vi "XML-RPC Server.vi"() -> ()   [LabVIEW 2014]
doc: "This VI is an XML-RPC Server - It will accept TCP/IP client connections, interpret a properly formatted XML-RPC request, launch the LabVIEW VI mapped to that request, and return the response in XML-RPC format to the requesting connection (client). VIs called by this server must be enclosed in a VI wrapper that supports conversion of the LV arguments in to XML-RPC format and converts the LV response to XML-RPC format.\n\nThis is a single-threaded server but it will handle multiple clients with some efficiency as connection requests are queued and the requested method is launched asynchronously so pending connections do not have to wait on a previous method request to complete unless the pending connection is trying to use a method already in progress.\n\nLicense\n\nThis work is licensed under the Creative Commons Attribution 3.0 Unported License. To view a copy of this license, visit http://creativecommons.org/licenses/by/3.0/ or send a letter to Creative Commons, 171 Second Street, Suite 300, San Francisco, California, 94105, USA.\n\nMark E. Smith, Sandia National Laboratories"
uses:
  Controls/methodCall.ctl
  Controls/methodResponse.ctl
  Controls/XML-RPC Server.ctl
panel:
  out "error log file path":path
  out "method path":path
  out "Parameters":string[](array[string])
  out "error out":errorcluster
  out "methodName":string
  in  "port":u16=8080
  in  "Private Data":T3={"error"={"status"=FALSE, "code"=0, "source"=""}, "active connection ID"=refnum, "methodCall"={"methodName"="", "Parameters"=[], "connection ID"=refnum}, "methodCall queue"=refnum, "methodResponse"={"value"="", "connection ID"=refnum}, "methodResponse queue"=refnum, "Error Log File Path"=path "", "Error Log Enabled"=FALSE, "Front Panel Window:State"=enum."Hidden"}
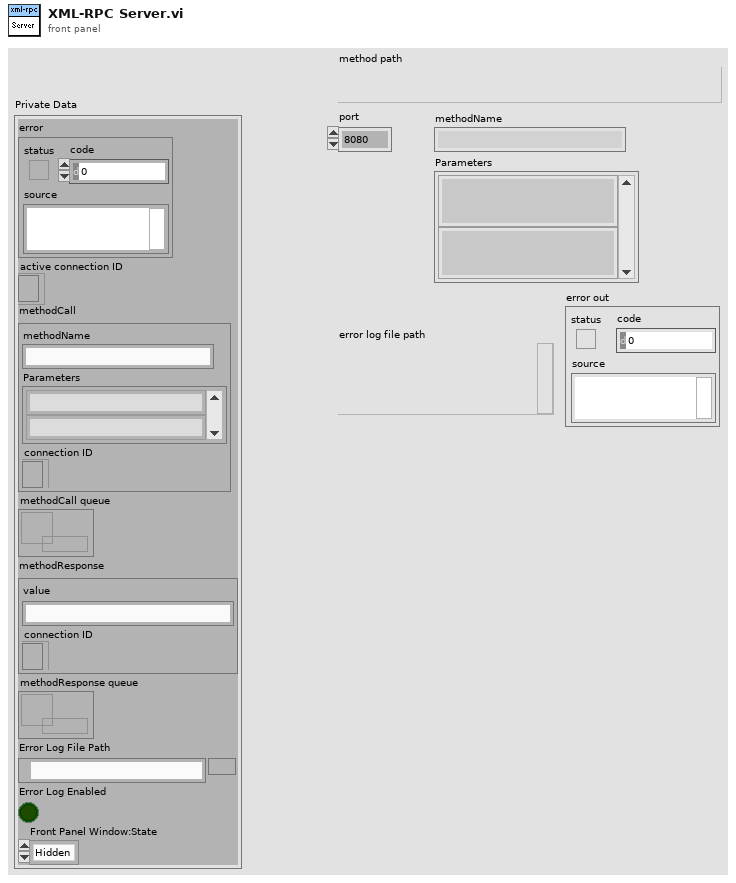
[diagram p1: front panel]
types:
  T1 = typedef "methodCall.ctl" = cluster{"methodName":string, "Parameters":string[], "connection ID":refnum<k5>}
  T2 = typedef "methodResponse.ctl" = cluster{"value":string, "connection ID":refnum<k5>}
  T3 = cluster{"error":errorcluster, "active connection ID":refnum<k5>, "methodCall":T1, "methodCall queue":refnum<queue>, "methodResponse":T2, "methodResponse queue":refnum<queue>, "Error Log File Path":path, "Error Log Enabled":bool, "Front Panel Window:State":enum32{"Invalid", "Standard", "Closed", "Hidden", "Minimized", "Maximized"}}
  T4 = typedef "XML-RPC Server.ctl" = enum16{"Initialize", "Dequeue", "Remote Procedure Call", "Server State", "Error", "Exit"}
  T5 = enum32{"Invalid", "Standard", "Closed", "Hidden", "Minimized", "Maximized"}
  T6 = enum32{"invalid app kind", "Development System", "Run Time System", "Student Edition", "Embedded LabVIEW", "Evaluation", "Custom"}
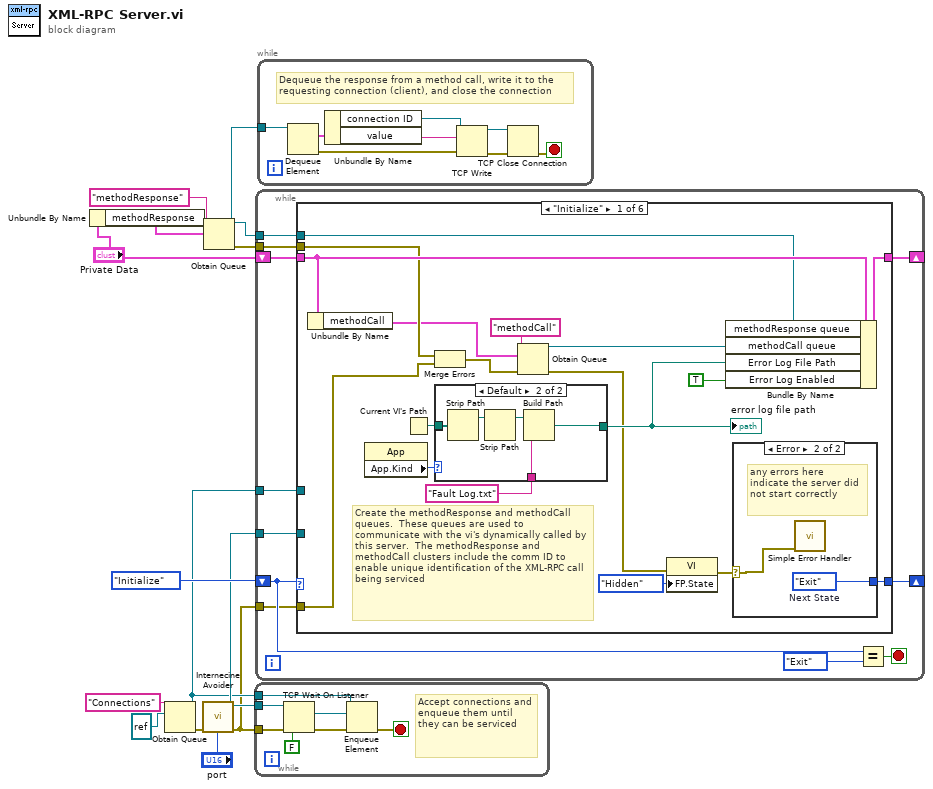
[diagram p0: block diagram]
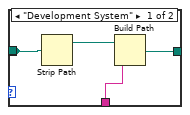
[diagram p2: hidden frame]
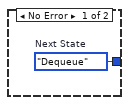
[diagram p3: hidden frame]
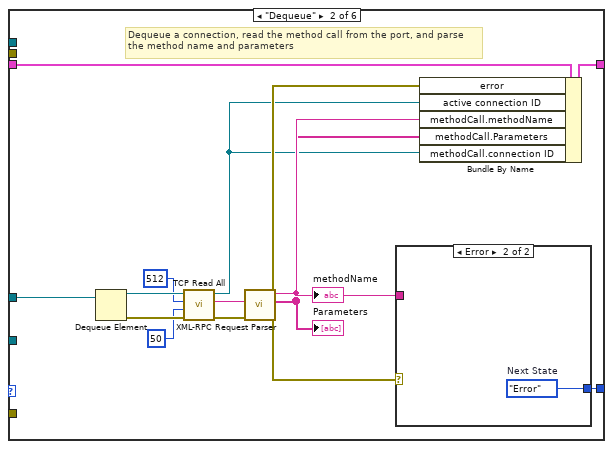
[diagram p4: hidden frame]
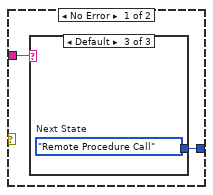
[diagram p5: hidden frame]
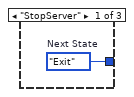
[diagram p6: hidden frame]
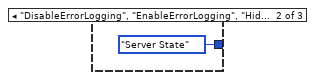
[diagram p7: hidden frame]
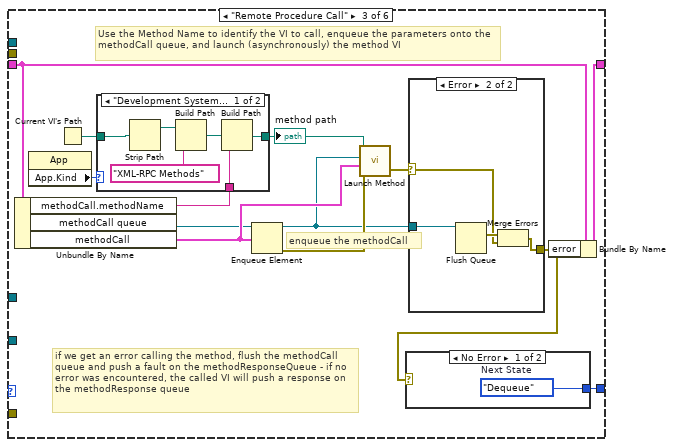
[diagram p8: hidden frame]
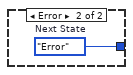
[diagram p9: hidden frame]
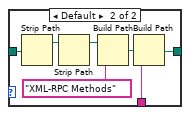
[diagram p11: hidden frame]
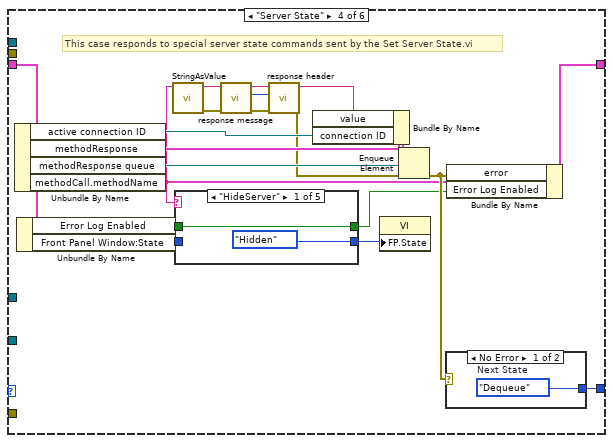
[diagram p12: hidden frame]
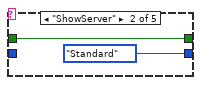
[diagram p13: hidden frame]
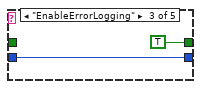
[diagram p14: hidden frame]
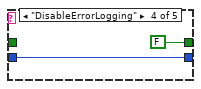
[diagram p15: hidden frame]
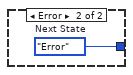
[diagram p17: hidden frame]
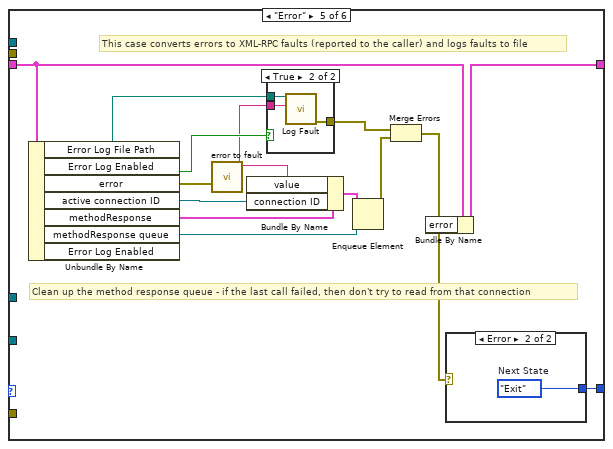
[diagram p18: hidden frame]
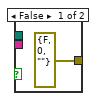
[diagram p19: hidden frame]
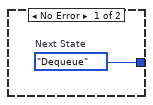
[diagram p20: hidden frame]
diagram:
  n1 = Unbundle By Name("Private Data") -> ("methodResponse"=w4:T2)
  n2 = Obtain Queue(name (unnamed)="Connections", element data type=refnum<k5> refnum ("listener ID out")) -> (queue out=w7:refnum<queue>, error out=w9:errorcluster)  [unwired: 3 in, 1 out]
  n3 = call <vilib>:"Internecine Avoider.vi"("Error In"=w9, "port"="port") -> ("error out"=w6:errorcluster, "connection ID"=w8:refnum<k5>)  [unwired: 8 in]
  n4 = Obtain Queue(name (unnamed)="methodResponse", element data type=w4) -> (queue out=w2:refnum<queue>, error out=w1:errorcluster)  [unwired: 3 in, 1 out]
  n5 = while {
    tunnel: w8 -> [w20]
    tunnel: w6 -> [w19]
    tunnel: w7 -> [w16]
    stop <- w14 stop-if-true
    # "Accept connections and enqueue them until they can be serviced"
    n6 = TCP Wait On Listener(8:w19, 10:FALSE ("resolve remote address (T)"), 11:w20) -> (0:w17:errorcluster, 4:w15:refnum<k5>)  [unwired: 1 in, 3 out]
    n7 = Enqueue Element(queue=w16, element=w15, error in (no error)=w17) -> (error out=w14:errorcluster)  [unwired: 1 in, 2 out]
  }
  n8 = while {
    shift-right: [w28] -> _
    shift-left: XML-RPC_Server."Initialize" ("Beginning State") -> [w29]
    shift-right: [w23] -> _
    shift-left: "Private Data" -> [w27]
    tunnel: w8 -> [w26]
    tunnel: w7 -> [w25]
    tunnel: w6 -> [w24]
    tunnel: w2 -> [w22]
    tunnel: w1 -> [w21]
    stop <- w31 stop-if-true
    n9 = case shown="\"Initialize\"" w29 {
      tunnel: [w49 w74 w92 w130 w156 XML-RPC_Server."Exit" ("Next State")] -> w28
      tunnel: w27 -> [w46 w73 w91 w119 w155 w172]
      tunnel: w26 -> [_ _ _ _ _ w173]
      tunnel: w25 -> [_ w75 _ _ _ _]
      tunnel: w24 -> [w41 _ _ _ _ _]
      tunnel: [w48 w72 w89 w128 w154 w172] -> w23
      tunnel: w22 -> [w44 _ _ _ _ _]
      tunnel: w21 -> [w43 _ _ _ _ _]
      frame "Initialize" {
        # "Create the methodResponse and methodCall queues.  These queues are used to communicate with the vi's dynamically called by this server.  The methodResponse and methodCall clusters include the comm ID to enable unique identification of the XML-RPC call being serviced"
        n10 = Unbundle By Name(w46) -> ("methodCall"=w42:T1)
        n11 = property class="App"() -> ("App.Kind"=w39:T6)  [unwired: 2 in, 2 out]
        n12 = Current VI's Path() -> (path=w38:path)
        n13 = Merge Errors(w43, w41) -> (w40:errorcluster)
        n14 = case shown="Default" w39 {
          tunnel: [w52 w56] -> _
          tunnel: [w53 w55] -> w36
          tunnel: w38 -> [w52 w56]
          tunnel: "Fault Log.txt" ("name or relative path") -> [w50 w54]
          frame "Development System" {
            n15 = Strip Path(path=w52) -> (stripped path=w51:path)  [unwired: 1 out]
            n16 = Build Path(base path=w51, name or relative path=w50) -> (appended path=w53:path)
          }
          frame Default {
            n17 = Strip Path(path=w56) -> (stripped path=w58:path)  [unwired: 1 out]
            n18 = Strip Path(path=w58) -> (stripped path=w57:path)  [unwired: 1 out]
            n19 = Build Path(base path=w57, name or relative path=w54) -> (appended path=w55:path)
          }
        }
        "error log file path" <- w36
        n20 = Obtain Queue(name (unnamed)="methodCall", element data type=w42, error in (no error)=w40) -> (queue out=w45:refnum<queue>, error out=w33:errorcluster)  [unwired: 2 in, 1 out]
        n21 = property class="VI"(error in=w33, "FP.State"=T5."Hidden" ("Front Panel Window:State")) -> (error out=w34:errorcluster)  [unwired: 1 in, 1 out]
        n22 = Bundle By Name(cluster=w46, "methodResponse queue"=w44, "methodCall queue"=w45, "Error Log File Path"=w36, "Error Log Enabled"=TRUE) -> (w48:T3)
        n23 = case shown="Error" w34 {
          selector: w34 -> [_ w60]
          tunnel: [w59 w61] -> w49
          frame No Error {
            w59 = XML-RPC_Server."Dequeue"  # Next State
          }
          frame Error {
            w61 = XML-RPC_Server."Exit"  # Next State
            # "any errors here indicate the server did not start correctly"
            n24 = call <vilib>:"Simple Error Handler.vi"("error in (no error)"=w60) -> ()  [unwired: 4 in, 5 out]
          }
        }
      }
      frame "Dequeue" {
        # "Dequeue a connection, read the method call from the port, and parse the method name and parameters"
        n25 = Dequeue Element(queue=w75) -> (element=w68:refnum<k5>, error out=w67:errorcluster)  [unwired: 2 in, 2 out]
        n26 = call "TCP Read All.vi"("error in"=w67, "TCP Timeout"=50 ("Timeout"), "Bytes Per Loop"=512, "connection ID in"=w68) -> ("error out"=w65:errorcluster, "data out"=w66:string, "connection ID out"=w62:refnum<k5>)  [unwired: 5 in]
        n27 = call "XML-RPC Request Parser.vi"("error in (no error)"=w65, "XML-RPC Call"=w66) -> ("error out"=w69:errorcluster, "Parameters"=w70:string[], "methodName"=w71:string)  [unwired: 7 in]
        "methodName" <- w71
        "Parameters" <- w70
        n28 = case shown="Error" w69 {
          tunnel: [w76 w81] -> w74
          tunnel: w71 -> [w77 _]
          frame No Error {
            n29 = case shown="Default" w77 {
              tunnel: [w78 XML-RPC_Server."Server State" ("Next State") w80] -> w76
              frame "StopServer" {
                w78 = XML-RPC_Server."Exit"  # Next State
              }
              frame "DisableErrorLogging", "EnableErrorLogging", "HideServer", "ShowServer" {
              }
              frame Default {
                w80 = XML-RPC_Server."Remote Procedure Call"  # Next State
              }
            }
          }
          frame Error {
            w81 = XML-RPC_Server."Error"  # Next State
          }
        }
        n30 = Bundle By Name(cluster=w73, "error"=w69, "active connection ID"=w62, "methodCall.methodName"=w71, "methodCall.Parameters"=w70, "methodCall.connection ID"=w62) -> (w72:T3)
      }
      frame "Remote Procedure Call" {
        # "Use the Method Name to identify the VI to call, enqueue the parameters onto the methodCall queue, and launch (asynchronously) the method VI"
        # "if we get an error calling the method, flush the methodCall queue and push a fault on the methodResponseQueue - if no error was encountered, the called VI will push a response on the methodResponse queue"
        # "enqueue the methodCall"
        n31 = Unbundle By Name(w91) -> ("methodCall.methodName"=w88:string, "methodCall queue"=w83:refnum<queue>, "methodCall"=w84:T1)
        n32 = property class="App"() -> ("App.Kind"=w93:T6)  [unwired: 2 in, 2 out]
        n33 = Current VI's Path() -> (path=w94:path)
        n34 = case shown="\"Development System\"" w93 {
          tunnel: w94 -> [w107 w114]
          tunnel: w88 -> [w103 w111]
          tunnel: [w102 w110] -> w85
          frame "Development System" {
            n35 = Strip Path(path=w107) -> (stripped path=w106:path)  [unwired: 1 out]
            n36 = Build Path(base path=w106, name or relative path="XML-RPC Methods") -> (appended path=w104:path)
            n37 = Build Path(base path=w104, name or relative path=w103) -> (appended path=w102:path)
          }
          frame Default {
            n38 = Strip Path(path=w114) -> (stripped path=w109:path)  [unwired: 1 out]
            n39 = Strip Path(path=w109) -> (stripped path=w108:path)  [unwired: 1 out]
            n40 = Build Path(base path=w108, name or relative path="XML-RPC Methods") -> (appended path=w112:path)
            n41 = Build Path(base path=w112, name or relative path=w111) -> (appended path=w110:path)
          }
        }
        "method path" <- w85
        n42 = Enqueue Element(queue=w83, element=w84) -> (queue out=w82:refnum<queue>, error out=w86:errorcluster)  [unwired: 2 in, 1 out]
        n43 = call "Launch Method.vi"("error in (no error)"=w86, "methodCall"=w84, "methodCall queue"=w82, "vi path"=w85) -> ("error out"=w87:errorcluster)  [unwired: 7 in]
        n44 = case shown="Error" w87 {
          selector: w87 -> [w97 w98]
          tunnel: [w97 w100] -> w90
          tunnel: w82 -> [_ w101]
          frame No Error {
          }
          frame Error {
            n45 = Flush Queue(queue=w101) -> (error out=w99:errorcluster)  [unwired: 1 in, 2 out]
            n46 = Merge Errors(w99, w98) -> (w100:errorcluster)
          }
        }
        n47 = case shown="No Error" w90 {
          tunnel: [w95 w96] -> w92
          frame No Error {
            w95 = XML-RPC_Server."Dequeue"  # Next State
          }
          frame Error {
            w96 = XML-RPC_Server."Error"  # Next State
          }
        }
        n48 = Bundle By Name(cluster=w91, "error"=w90) -> (w89:T3)
      }
      frame "Server State" {
        # "This case responds to special server state commands sent by the Set Server State.vi"
        n49 = Unbundle By Name(w119) -> ("active connection ID"=w133:refnum<k5>, "methodResponse"=w134:T2, "methodResponse queue"=w131:refnum<queue>, "methodCall.methodName"=w127:string)
        n50 = Unbundle By Name(w119) -> ("Error Log Enabled"=w118:bool, "Front Panel Window:State"=w117:T5)
        n51 = call "StringAsValue.vi"("scalar value (string)"=w127) -> ("error out"=w125:errorcluster, "scalar string"=w126:string)  [unwired: 9 in]
        n52 = case shown="\"HideServer\"" w127 {
          tunnel: w118 -> [w135 w137 _ _ w144]
          tunnel: w117 -> [_ _ w140 w142 w143]
          tunnel: [T5."Hidden" ("Front Panel Window:State") T5."Standard" ("Front Panel Window:State") w140 w142 w143] -> w116
          tunnel: [w135 w137 TRUE ("Error Log Enabled") FALSE ("Error Log Enabled") w144] -> w115
          frame "HideServer" {
          }
          frame "ShowServer" {
          }
          frame "EnableErrorLogging" {
          }
          frame "DisableErrorLogging" {
          }
          frame Default {
            # "Do Nothing"
          }
        }
        n53 = call "response message.vi"("error in"=w125, "params (formatted)"=w126) -> ("error out"=w122:errorcluster, "length"=w124:i32, "response"=w123:string)  [unwired: 7 in]
        n54 = call "response header.vi"("error in"=w122, "Content-Length"=w124, "Content String"=w123) -> ("error out"=w120:errorcluster, "response string"=w121:string)  [unwired: 7 in]
        n55 = Bundle By Name(cluster=w134, "value"=w121, "connection ID"=w133) -> (w132:T2)
        n56 = property class="VI"("FP.State"=w116) -> ()  [unwired: 2 in, 2 out]
        n57 = Enqueue Element(queue=w131, element=w132, error in (no error)=w120) -> (error out=w129:errorcluster)  [unwired: 1 in, 2 out]
        n58 = case shown="No Error" w129 {
          tunnel: [w145 w146] -> w130
          frame No Error {
            w145 = XML-RPC_Server."Dequeue"  # Next State
          }
          frame Error {
            w146 = XML-RPC_Server."Error"  # Next State
          }
        }
        n59 = Bundle By Name(cluster=w119, "error"=w129, "Error Log Enabled"=w115) -> (w128:T3)
      }
      frame "Error" {
        # "Clean up the method response queue - if the last call failed, then don't try to read from that connection"
        # "This case converts errors to XML-RPC faults (reported to the caller) and logs faults to file"
        n60 = Unbundle By Name(w155) -> ("Error Log File Path"=w153:path, "Error Log Enabled"=w151:bool, "error"=w152:errorcluster, "active connection ID"=w159:refnum<k5>, "methodResponse"=w160:T2, "methodResponse queue"=w157:refnum<queue>)  [unwired: 1 out]
        n61 = call "error to fault.vi"("error cluster"=w152) -> ("response string"=w150:string)  [unwired: 10 in]
        n62 = Bundle By Name(cluster=w160, "value"=w150, "connection ID"=w159) -> (w158:T2)
        n63 = case shown="True" w151 {
          tunnel: w153 -> [_ w164]
          tunnel: w150 -> [_ w163]
          tunnel: [errorcluster {"status"=FALSE, "code"=0, "source"=""} ("error out") w162] -> w149
          frame False {
          }
          frame True {
            n64 = call "Log Fault.vi"("Error String"=w163, "Path In"=w164) -> ("error out"=w162:errorcluster)  [unwired: 9 in]
          }
        }
        n65 = Enqueue Element(queue=w157, element=w158) -> (error out=w148:errorcluster)  [unwired: 2 in, 2 out]
        n66 = Merge Errors(w149, w148) -> (w147:errorcluster)
        n67 = Bundle By Name(cluster=w155, "error"=w147) -> (w154:T3)
        n68 = case shown="Error" w147 {
          tunnel: [w165 w166] -> w156
          frame No Error {
            w165 = XML-RPC_Server."Dequeue"  # Next State
          }
          frame Error {
            w166 = XML-RPC_Server."Exit"  # Next State
          }
        }
      }
      frame "Exit" {
        # "close the listener"
        # "release the response queue"
        n69 = Unbundle By Name(w172) -> ("methodResponse queue"=w171:refnum<queue>)
        n70 = Release Queue(queue=w171) -> (error out=w170:errorcluster)  [unwired: 2 in, 2 out]
        n71 = TCP Close Connection(connection ID=w173) -> (error out=w169:errorcluster)  [unwired: 2 in, 1 out]
        n72 = property class="App"() -> ("App.Kind"=w168:T6)  [unwired: 2 in, 2 out]
        n73 = case shown="Default" w168 {
          tunnel: w170 -> [_ _]
          tunnel: w169 -> [_ _]
          frame Default {
            n74 = property class="VI"("Front Panel.Open"=FALSE ("Front Panel Window:Open")) -> ()  [unwired: 2 in, 2 out]
          }
          frame "Development System" {
          }
        }
        n75 = Unbundle By Name(w172) -> ("error"=→"error out":errorcluster)
      }
    }
    n76 = Equal?(x=w29, y=XML-RPC_Server."Exit" ("States")) -> (x = y?=w31:bool)
  }
  n77 = while {
    tunnel: w2 -> [w176]
    stop <- w177 stop-if-true
    # "Dequeue the response from a method call, write it to the requesting connection (client), and close the connection"
    n78 = Dequeue Element(queue=w176) -> (element=w182:T2, error out=w181:errorcluster)  [unwired: 2 in, 2 out]
    n79 = Unbundle By Name(w182) -> ("connection ID"=w178:refnum<k5>, "value"=w183:string)
    n80 = TCP Write(connection ID=w178, data in=w183, error in (no error)=w181) -> (connection ID out=w179:refnum<k5>, error out=w180:errorcluster)  [unwired: 1 in, 1 out]
    n81 = TCP Close Connection(connection ID=w179, error in (no error)=w180) -> (error out=w177:errorcluster)  [unwired: 1 in, 1 out]
  }
